vi "LOGIC_Compute.vi"(0 "Database RefNum in":T1, 1 "log_file":path, 5 "expstart":bool, 7 "readstart":bool, 9 "readend":bool, 11 "error in (no error)":errorcluster, 12 "raw bpp":i32=16, 13 "usc_tmout in":i32) -> (6 "orig name":string, 8 "usc_tmout":i32, 10 "created":bool, 15 "error out":errorcluster)   [LabVIEW 2016]
uses:
  DBSHAND/private/vis/DatabaseHand_RefNum.ctl
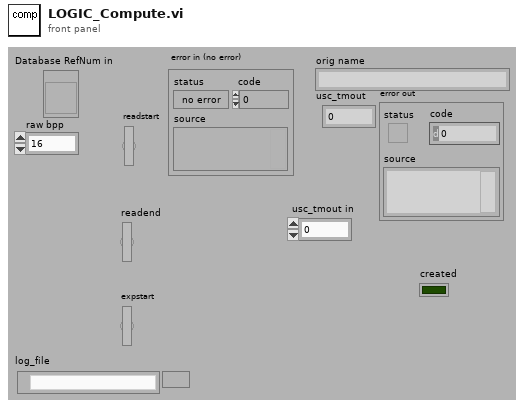
[diagram p1: front panel]
types:
  T1 = typedef "DatabaseHand_RefNum.ctl" = refnum<vi>
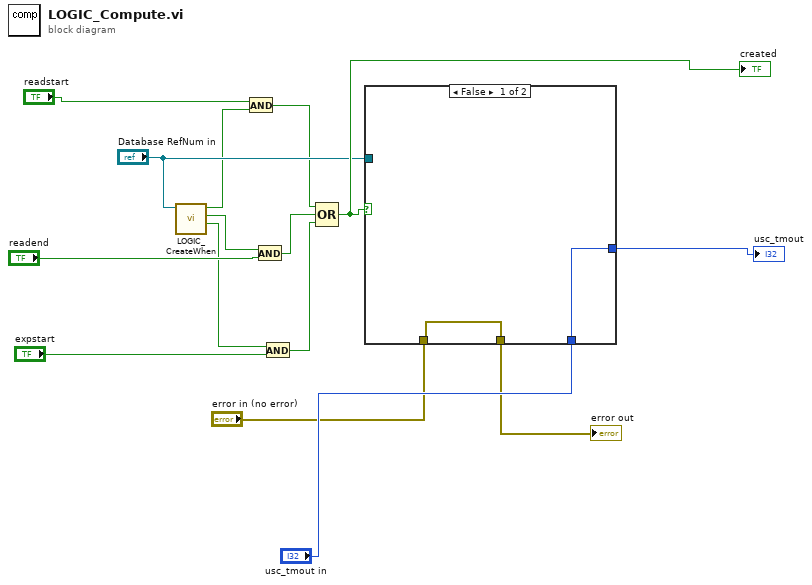
[diagram p0: block diagram]
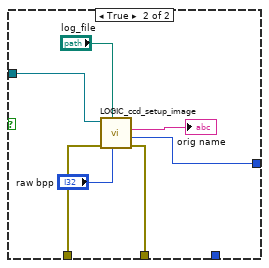
[diagram p2: hidden frame]
diagram:
  n1 = call "LOGIC_CreateWhen.vi"("Database RefNum in"="Database RefNum in") -> ("onexpstart"=w5:bool, "onreadend"=w7:bool, "onreadstart"=w8:bool)  [unwired: 8 out]
  n2 = And(x="readstart", y=w8) -> (x .and. y?=w3:bool)
  n3 = And(x=w7, y="readend") -> (x .and. y?=w2:bool)
  n4 = And(x=w5, y="expstart") -> (x .and. y?=w1:bool)
  n5 = Compound Arithmetic op=OR(w3, w2, w1) -> (w15:bool)
  "created" <- w15
  n6 = case shown="False" w15 {
    tunnel: "error in (no error)" -> [w17 w24]
    tunnel: "Database RefNum in" -> [_ w23]
    tunnel: [w17 w19] -> w10
    tunnel: [w16 w18] -> w13
    tunnel: "usc_tmout in" -> [w16 _]
    frame False {
    }
    frame True {
      n7 = call "LOGIC_ccd_setup_image.vi"("raw bpp"="raw bpp", "log_file"="log_file", "error in (no error)"=w24, "Database RefNum in"=w23) -> ("error out"=w19:errorcluster, "usc_tmout"=w18:i32, "orig name"=→"orig name":string)  [unwired: 5 out]
    }
  }
  "usc_tmout" <- w13
  "error out" <- w10
